vi "DAQ.Write.vi"(8 "error in (no error)":errorcluster, 10 "Write":T1, 11 "DAQmx.AO in":refnum<class "DAQmx.AO.lvclass">) -> (0 "error out":errorcluster, 3 "DAQmx.AO out":refnum<class "DAQmx.AO.lvclass">)   [LabVIEW 2016, in "DAQmx.AO.lvclass"]
uses:
  DAQmx.AO.lvclass
  C:/user/patrick/hg/lockin.SMO/lvsrc/DAQ/DAQ.lvclass
  C:/user/patrick/hg/lockin.SMO/lvsrc/DAQmx/DAQmx.lvclass
  DAQ/Typedefs/PrivateEvents--DAQ.Write.ctl
  DAQ/DAQ.lvclass
  DAQmx/DAQmx.lvclass
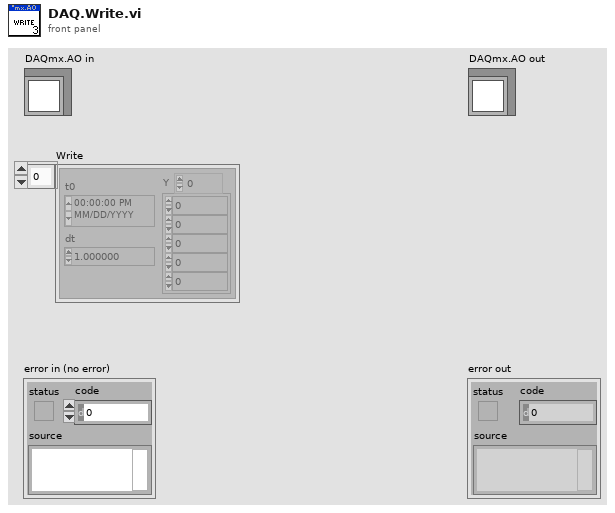
[diagram p1: front panel]
types:
  T1 = typedef "DAQ.lvclass/PrivateEvents--DAQ.Write.ctl" = waveform(dbl)[]
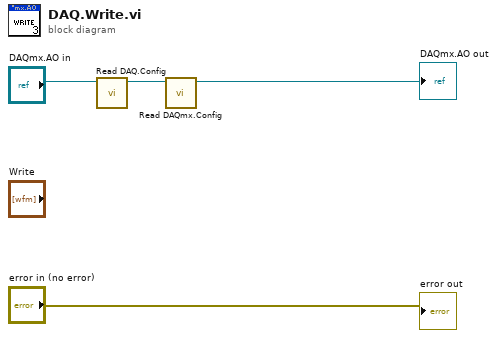
[diagram p0: block diagram]
diagram:
  n1 = call "Read DAQ.Config.vi"("DAQ in"="DAQmx.AO in") -> ("DAQ out"=w4:refnum<class "DAQmx.AO.lvclass">)  [unwired: 8 in, 2 out]
  n2 = call "Read DAQmx.Config.vi"("DAQmx in"=w4) -> ("DAQmx out"=→"DAQmx.AO out":refnum<class "DAQmx.AO.lvclass">)  [unwired: 8 in, 2 out]
  "error out" <- "error in (no error)"
